vi "DigitalOutput.vi"(8 "Array in":bool[](array[boolean])=[FALSE, FALSE, FALSE, FALSE, FALSE, FALSE, FALSE, FALSE], 10 "Digital Output":bool, 11 "Output Channel":T1(ring)) -> (0 "Updated array out":bool[](array[boolean]))   [LabVIEW 2025]
panel:
  # "Write single digital output to output array\n\nInserts digital output value into digital output \narray in preperation for write to MB server.\nIf output array input is unwired, output array\nis initialised as 8x1 array of type bool.\n\nINPUTS:\n  1. Discrete output channel -- int 0-7 or auto\n      configured enum DO-0 -> DO-7\n   2. Array of values to write to MB server.\n       bool array with dimension 8x1\n\nOUTPUTS:\n   1. Array of values to write to MB server\n       bool with dimension 8x1. -- updated array\n       obtained from input 2"
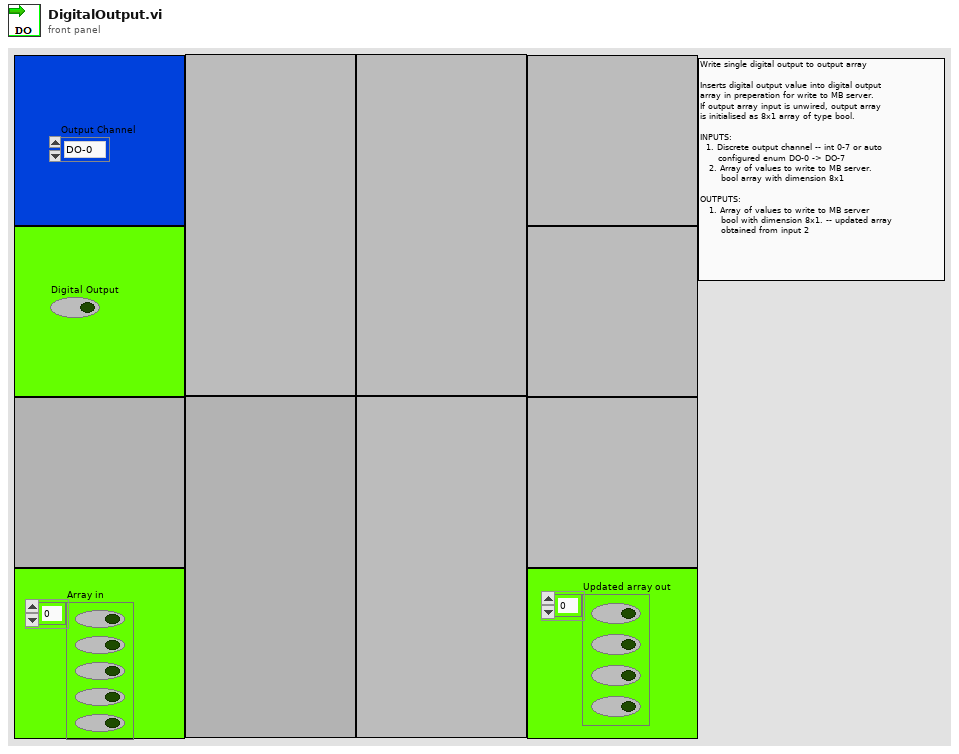
[diagram p1: front panel]
types:
  T1 = enum16{"DO-0", "DO-1", "DO-2", "DO-3", "DO-4", "DO-5", "DO-6", "DO-7"}
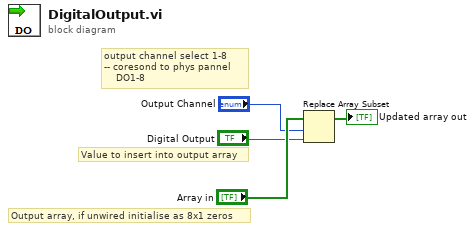
[diagram p0: block diagram]
diagram:
  # "Output array, if unwired initialise as 8x1 zeros"
  # "Value to insert into output array"
  # "output channel select 1-8\n-- coresond to phys pannel\n    DO1-8"
  n1 = Replace Array Subset(array="Array in", new element="Digital Output", index="Output Channel") -> (→"Updated array out":bool[])
